vi "PH_Synchrolock_Watch.initialize GUI.vi"(0 "i ref in":refnum<vi>, 5 "error in (no error)":errorcluster) -> (14 "i ref out":refnum<vi>, 19 "error out":errorcluster)   [LabVIEW 2014, in "PH_Synchrolock_Watch.lvlib"]
doc: "In this VI own attributes are set as well as GUI elements."
uses:
  PH_Synchrolock_Watch.lvlib
  PH_Basics/PH_Common/PH_Common.lvlib
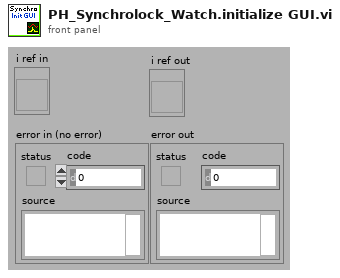
[diagram p1: front panel]
types:
  T1 = typedef "PH_Synchrolock_Watch.lvlib/PH_Synchrolock_Watch.i attribute.ctl" = cluster{"GUI Refs":cluster{"Mean Phase Graph":refnum<vi>, "RF Amplitude Graph":refnum<vi>, "Mira Amplitude Graph":refnum<vi>, "MIRA State":refnum<vi>, "Mean Phase":refnum<vi>, "RF Amplitude":refnum<vi>, "Mira Amplitude":refnum<vi>, "Mean Phase in range?":refnum<vi>, "RF Amplitude above limit?":refnum<vi>, "Mira Amplitude in range?":refnum<vi>, "Mean phase upper limit":refnum<vi>, "Mean phase lower limit":refnum<vi>, "RF Amplitude lower limit":refnum<vi>, "Mira Amplitude lower limit":refnum<vi>, "Mira Amplitude upper limit":refnum<vi>, "Waveform End":refnum<vi>, "Mira scope":refnum<vi>, "Reset Mira warning":refnum<vi>}, "Status":cluster{"Reset Warning":bool}, "Mean Phase":cluster{"Current Value":dbl, "Upper Limit":dbl, "Lower Limit":dbl, "Data":cluster{dbl[], dbl[]}}, "RF":cluster{"Current Value":dbl, "Lower Limit":dbl, "Data":cluster{dbl[], dbl[]}}, "MIRA":cluster{"Current Value":dbl, "Upper Limit":dbl, "Lower Limit":dbl, "Data":cluster{dbl[], dbl[]}}, "Waveform End":i32}
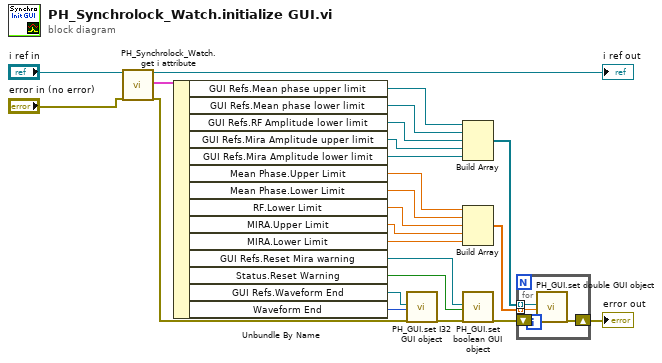
[diagram p0: block diagram]
diagram:
  n1 = call "PH_Synchrolock_Watch.get i attribute.vi"("i ref in"="i ref in", "error in (no error)"="error in (no error)") -> ("i ref out"=→"i ref out":refnum<vi>, "i attribute"=w21:T1, "error out"=w23:errorcluster)  [unwired: 15 in]
  n2 = Unbundle By Name(w21) -> ("GUI Refs.Mean phase upper limit"=w10:refnum<vi>, "GUI Refs.Mean phase lower limit"=w11:refnum<vi>, "GUI Refs.RF Amplitude lower limit"=w12:refnum<vi>, "GUI Refs.Mira Amplitude upper limit"=w13:refnum<vi>, "GUI Refs.Mira Amplitude lower limit"=w14:refnum<vi>, "Mean Phase.Upper Limit"=w5:dbl, "Mean Phase.Lower Limit"=w6:dbl, "RF.Lower Limit"=w7:dbl, "MIRA.Upper Limit"=w8:dbl, "MIRA.Lower Limit"=w9:dbl, "GUI Refs.Reset Mira warning"=w16:refnum<vi>, "Status.Reset Warning"=w17:bool, "GUI Refs.Waveform End"=w20:refnum<vi>, "Waveform End"=w19:i32)
  n3 = call "PH_GUI.set I32 GUI object.vi"("I32 GUI Ref"=w20, "value"=w19, "error in (no error)"=w23) -> ("error out"=w18:errorcluster)  [unwired: 16 in]
  n4 = Build Array(w10, w11, w12, w13, w14) -> (w3:refnum<vi>[])
  n5 = Build Array(w5, w6, w7, w8, w9) -> (w4:dbl[])
  n6 = call "PH_GUI.set boolean GUI object.vi"("Boolean Knob GUI Ref"=w16, "Value"=w17, "error in (no error)"=w18) -> ("error out"=w15:errorcluster)  [unwired: 16 in]
  n7 = for {
    shift-right: [w27] -> w1
    shift-left: w15 -> [w28]
    tunnel: w4 -> [w26] mode=indexing
    tunnel: w3 -> [w25] mode=indexing
    n8 = call "PH_GUI.set double GUI object.vi"("GUI object Ref"=w25, "value"=w26, "error in (no error)"=w28) -> ("error out"=w27:errorcluster)  [unwired: 16 in]
  }
  "error out" <- w1
